vi "PWM_REF.vi"() -> ()   [LabVIEW 2015]
uses:
  <vilib>/myRIO/Instrument Drivers/Onboard IO/PWM/typedefs/PWM Reference.ctl
  <vilib>/myRIO/Common/Instrument Driver Framework/Utilities/typedefs/myRIO Generic Hardware Reference.ctl
  <vilib>/myRIO/Common/Instrument Driver Framework/Utilities/typedefs/Hardware Version Enum.ctl
  <vilib>/myRIO/Common/Instrument Driver Framework/Utilities/typedefs/myRIO v1.0 Reference.ctl
  <vilib>/myRIO/Common/Instrument Driver Framework/Utilities/typedefs/Generic FPGA Reference.ctl
  <vilib>/myRIO/Common/Instrument Driver Framework/myRIO v1.0/PWM/typedefs/PWM Channels Enum.ctl
  <vilib>/myRIO/Instrument Drivers/Onboard IO/PWM/typedefs/PWM Configuration.ctl
  <vilib>/userdefined/High Color/nirio_resource_hc.ctl
  <vilib>/myRIO/Common/Instrument Driver Framework/myRIO v1.0/PWM/vis/myRIO v1.1 Open PWM.vi
  <vilib>/myRIO/Common/Instrument Driver Framework/Utilities/vis/Validate Channels.vi
  <vilib>/myRIO/Common/Instrument Driver Framework/myRIO v1.0/PWM/vis/myRIO v1.0 Reserve PWM.vi
  <vilib>/myRIO/Common/Instrument Driver Framework/myRIO v1.0/PWM/vis/myRIO v1.0 Close PWM.vi
  <vilib>/myRIO/Common/Instrument Driver Framework/myRIO v1.0/PWM/vis/myRIO v1.0 Build MUX Configuration PWM.vi
  <vilib>/myRIO/Common/Instrument Driver Framework/myRIO v1.0/Resource Manager/vis/myRIO v1.0 Reserve Channel List.vi
  <vilib>/myRIO/Common/Instrument Driver Framework/myRIO v1.0/PWM/vis/myRIO v1.0 Unreserve PWM.vi
  <vilib>/myRIO/Common/Instrument Driver Framework/myRIO v1.0/Resource Manager/vis/myRIO v1.0 Create Configuration List.vi
  <vilib>/myRIO/Common/Instrument Driver Framework/myRIO v1.0/Resource Manager/vis/myRIO v1.0 Reserve Channel.vi
  <vilib>/myRIO/Common/Instrument Driver Framework/myRIO v1.0/Resource Manager/vis/myRIO v1.0 Unreserve Channel.vi
  <vilib>/myRIO/Common/Instrument Driver Framework/myRIO v1.0/Resource Manager/vis/myRIO v1.0 Unreserve Channel List.vi
  <vilib>/myRIO/Common/Instrument Driver Framework/myRIO v1.0/Resource Manager/vis/myRIO v1.0 Build Mutex Name.vi
  <vilib>/Utility/VariantDataType/GetNumericInfo.vi
  <vilib>/Utility/error.llb/Error Cluster From Error Code.vi
  <vilib>/myRIO/Common/Instrument Driver Framework/myRIO v1.0/myRIO v1.1 Open.vi
  <vilib>/myRIO/Common/Instrument Driver Framework/Utilities/vis/IO Manager.vi
  <vilib>/myRIO/Common/Instrument Driver Framework/Utilities/vis/Configuration Manager.vi
  <vilib>/myRIO/Common/Instrument Driver Framework/myRIO v1.0/Resource Manager/vis/myRIO v1.0 Configure IO.vi
  <vilib>/myRIO/Common/Instrument Driver Framework/myRIO v1.0/myRIO v1.0 Close.vi
  <vilib>/myRIO/Common/Instrument Driver Framework/myRIO v1.0/PWM/vis/myRIO v1.0 Write PWM.vi
  <vilib>/myRIO/Common/Instrument Driver Framework/myRIO v1.0/PWM/vis/myRIO v1.0 Shutdown PWM.vi
  <vilib>/myRIO/Instrument Drivers/Onboard IO/PWM/vis/myRIO PWM Open.xnode
  <vilib>/myRIO/Instrument Drivers/Onboard IO/PWM/PWM.lvlib
panel:
  in  "Tab Control":enum32{"Duty Cycle Controller"}(tab)
  in  "Frequency [Hz]":dbl(slide)=1000.0 scale=40.0..40000.0
  in  "Base Bladder Inlet":dbl(slide)=1.0 scale=0.0..1.0
  in  "PWM 2":tag="A/PWM2"
  in  "PWM 0":tag="A/PWM0"
  in  "B/PWM 2":tag="B/PWM2"
  in  "PWM 1":tag="A/PWM1"
  in  "Right Bladder Inlet":dbl(slide)=0.5 scale=0.0..1.0
  in  "Base Bladder Outlet":dbl(slide)=0.5 scale=0.0..1.0
  in  "Left Bladder Inlet":dbl(slide)=0.5 scale=0.0..1.0
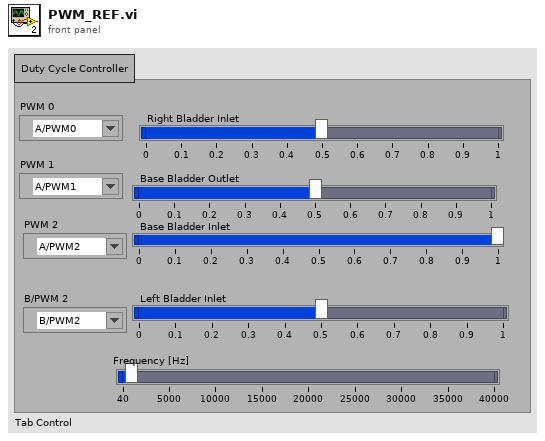
[diagram p1: front panel]
types:
  T1 = typedef "PWM.lvlib/PWM Reference.ctl" = cluster{"myRIO Reference":T2, "PWM Channels Enum":T6, "PWM Configuration":T7}
  T2 = typedef "myRIO Generic Hardware Reference.ctl" = cluster{"myRIO Model":T3, "myRIO Hardware Reference":T4}
  T3 = typedef "Hardware Version Enum.ctl" = enum16{"Unknown", "myRIO-1900", "myRIO-1950", "roboRIO"}
  T4 = typedef "myRIO v1.0 Reference.ctl" = cluster{"Generic FPGA Reference":T5, "Allow multiple opens":bool}
  T5 = typedef "Generic FPGA Reference.ctl" = refnum<k20>
  T6 = typedef "PWM Channels Enum.ctl" = enum16{"Not Connected", "C/PWM0", "C/PWM1", "A/PWM0", "A/PWM1", "A/PWM2", "B/PWM0", "B/PWM1", "B/PWM2", "PWM/PWM0", "PWM/PWM1", "PWM/PWM2", "PWM/PWM3", "PWM/PWM4", "PWM/PWM5", "PWM/PWM6", "PWM/PWM7", "PWM/PWM8", "PWM/PWM9"}
  T7 = typedef "PWM.lvlib/PWM Configuration.ctl" = cluster{"Frequency":dbl, "Duty Cycle":dbl}
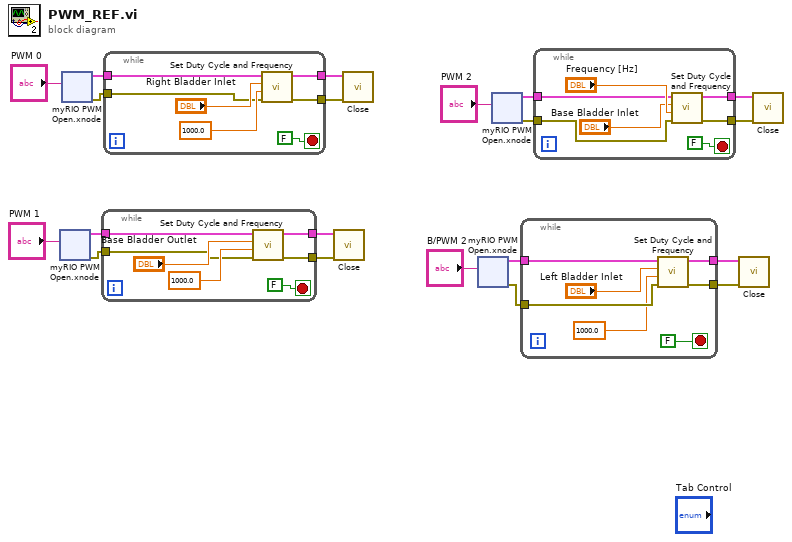
[diagram p0: block diagram]
diagram:
  n1 = xnode "myRIO PWM Open.xnode"("Channel Name"="PWM 1") -> ("error out"=w4:errorcluster, "PWM Ref Out"=w12:T1)  [unwired: 2 in]
  n2 = xnode "myRIO PWM Open.xnode"("Channel Name"="PWM 0") -> ("error out"=w2:errorcluster, "PWM Ref Out"=w15:T1)  [unwired: 2 in]
  n3 = while {
    tunnel: w12 -> [w26]
    tunnel: [w27] -> w11
    tunnel: [w22] -> w5
    tunnel: w4 -> [w21]
    stop <- FALSE stop-if-true
    n4 = call <vilib>:"Set Duty Cycle and Frequency.vi"("error in (no error)"=w21, "Frequency [Hz]"=1000.0, "Duty Cycle"="Base Bladder Outlet", "PWM Ref In"=w26) -> ("error out"=w22:errorcluster, "PWM Ref Out"=w27:T1)  [unwired: 5 in]
  }
  n5 = while {
    tunnel: w15 -> [w33]
    tunnel: [w34] -> w14
    tunnel: [w29] -> w3
    tunnel: w2 -> [w28]
    stop <- FALSE stop-if-true
    n6 = call <vilib>:"Set Duty Cycle and Frequency.vi"("error in (no error)"=w28, "Frequency [Hz]"=1000.0, "Duty Cycle"="Right Bladder Inlet", "PWM Ref In"=w33) -> ("error out"=w29:errorcluster, "PWM Ref Out"=w34:T1)  [unwired: 5 in]
  }
  n7 = call <vilib>:"Close.vi"("error in (no error)"=w5, "PWM Ref In"=w11) -> ()  [unwired: 9 in, 1 out]
  n8 = call <vilib>:"Close.vi"("error in (no error)"=w3, "PWM Ref In"=w14) -> ()  [unwired: 9 in, 1 out]
  n9 = xnode "myRIO PWM Open.xnode"("Channel Name"="B/PWM 2") -> ("error out"=w6:errorcluster, "PWM Ref Out"=w9:T1)  [unwired: 2 in]
  n10 = xnode "myRIO PWM Open.xnode"("Channel Name"="PWM 2") -> ("error out"=w1:errorcluster, "PWM Ref Out"=w20:T1)  [unwired: 2 in]
  n11 = while {
    tunnel: w9 -> [w39]
    tunnel: [w38] -> w8
    tunnel: [w37] -> w7
    tunnel: w6 -> [w36]
    stop <- FALSE stop-if-true
    n12 = call <vilib>:"Set Duty Cycle and Frequency.vi"("error in (no error)"=w36, "Frequency [Hz]"=1000.0, "Duty Cycle"="Left Bladder Inlet", "PWM Ref In"=w39) -> ("error out"=w37:errorcluster, "PWM Ref Out"=w38:T1)  [unwired: 5 in]
  }
  n13 = while {
    tunnel: [w47] -> w17
    tunnel: [w46] -> w18
    tunnel: w20 -> [w44]
    tunnel: w1 -> [w42]
    stop <- FALSE stop-if-true
    n14 = call <vilib>:"Set Duty Cycle and Frequency.vi"("error in (no error)"=w42, "Frequency [Hz]"="Frequency [Hz]", "Duty Cycle"="Base Bladder Inlet", "PWM Ref In"=w44) -> ("error out"=w46:errorcluster, "PWM Ref Out"=w47:T1)  [unwired: 5 in]
  }
  n15 = call <vilib>:"Close.vi"("error in (no error)"=w7, "PWM Ref In"=w8) -> ()  [unwired: 9 in, 1 out]
  n16 = call <vilib>:"Close.vi"("error in (no error)"=w18, "PWM Ref In"=w17) -> ()  [unwired: 9 in, 1 out]
